vi "PPSU Values 2.vi"(8 "error in":errorcluster, 11 "PPSU 2 Q":refnum<queue>) -> (0 "Fehler":errorcluster caption="Error out")   [LabVIEW 2022 SP3]
uses:
  6D_Global.vi
panel:
  out "Read data 3":string
  out "Read data (hex) 2":u8[](array[numeric]) format="%.0x"
  out "Read data 2":string
  out "Read data (hex)":u8[](array[numeric]) format="%.0x"
  out "Read data":string
  out "array 2":string[](array[string])
  out "match substring":string
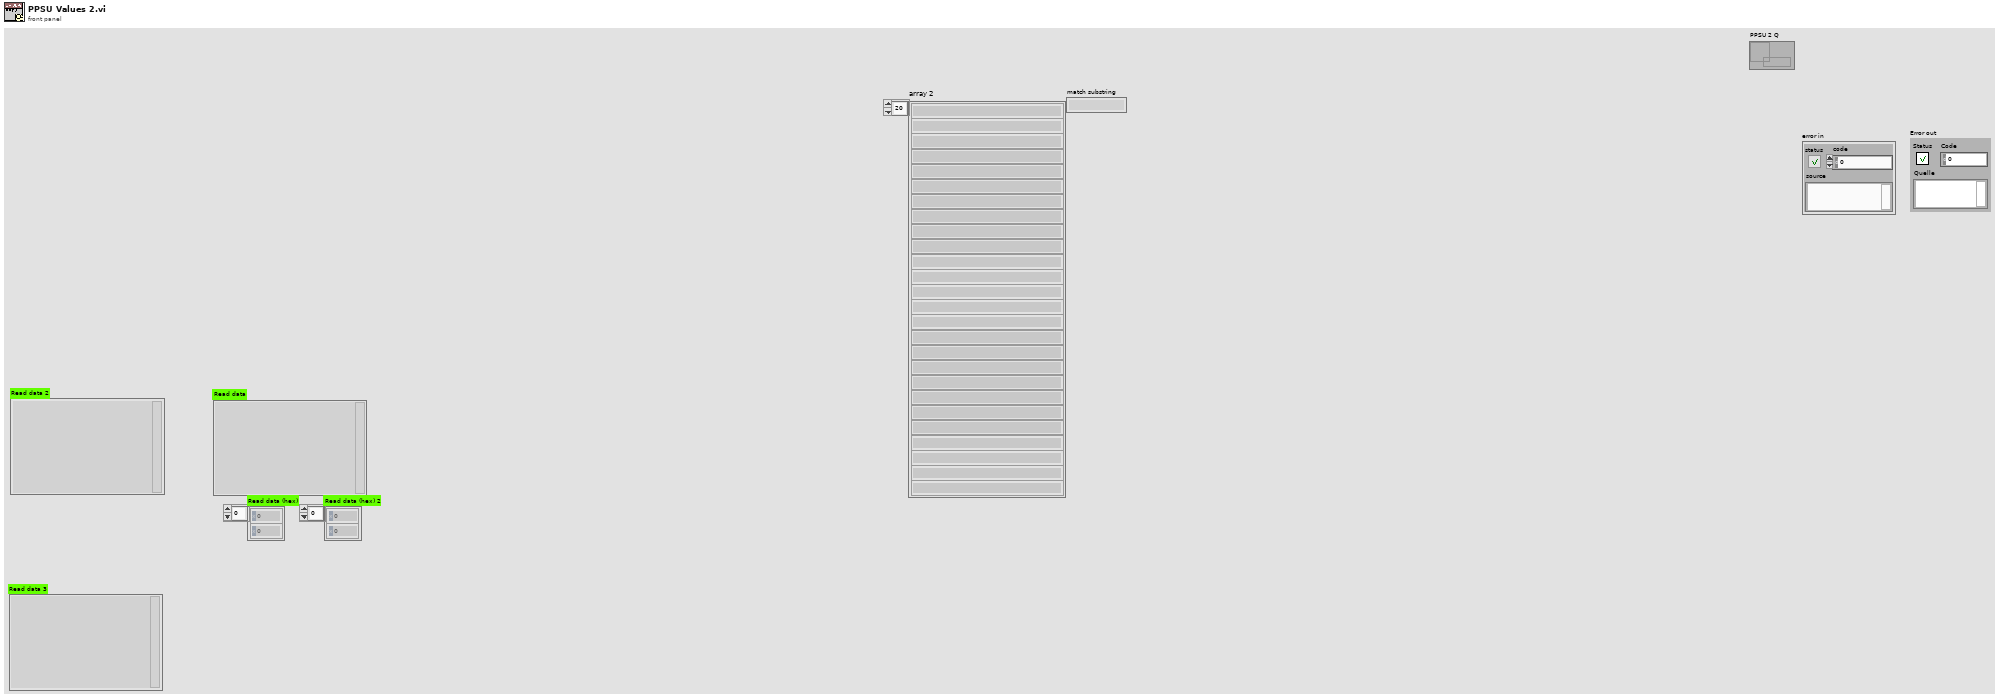
[diagram p1: front panel]
types:
  T1 = cluster{"Alarm":bool, "Power Fail":bool, "OVD":bool, "OCD":bool, "OPD":bool, "MSP":bool}
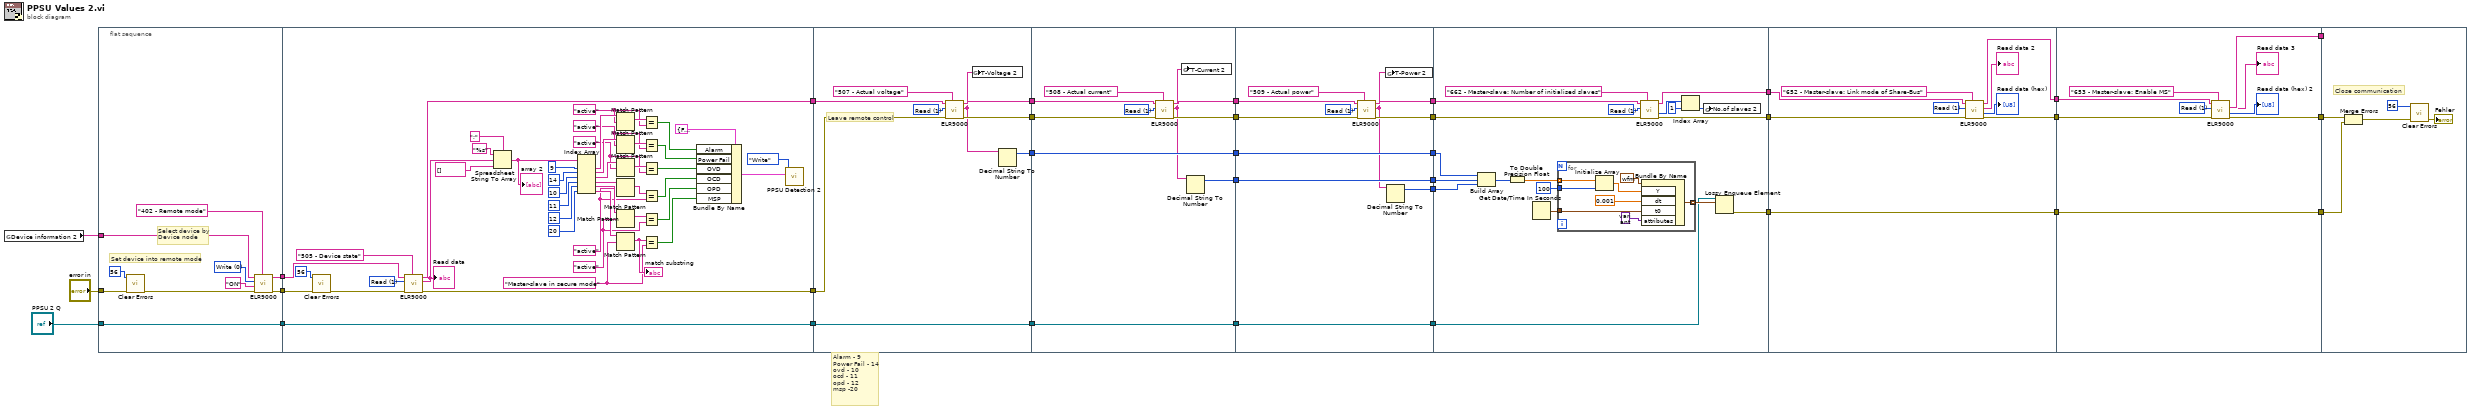
[diagram p0: block diagram]
diagram:
  # "Alarm - 9\nPower Fail - 14\novd - 10\nocd - 11\nopd - 12\nmsp -20"
  n1 = global read "6D_Global.vi" "Device information 2"() -> (w16:string[])
  n2 = flat-sequence {
    tunnel: [w43] -> w32
    tunnel: [w42] -> w33
    tunnel: w16 -> [w38]
    tunnel: "error in" -> [w36]
    tunnel: "PPSU 2 Q" -> [w34]
    tunnel: [w34] -> w14
    tunnel: [w90] -> w31
    tunnel: w33 -> [w87]
    tunnel: w32 -> [w86]
    tunnel: [w55] -> w30
    tunnel: w14 -> [w44]
    tunnel: [w44] -> w13
    tunnel: [w95] -> w29
    tunnel: w31 -> [w97]
    tunnel: [w96] -> w28
    tunnel: w30 -> [w94]
    tunnel: w13 -> [w93]
    tunnel: [w93] -> w12
    tunnel: [w91] -> w9
    tunnel: w29 -> [w105]
    tunnel: [w104] -> w27
    tunnel: w28 -> [w106]
    tunnel: [w107] -> w26
    tunnel: w12 -> [w103]
    tunnel: [w103] -> w11
    tunnel: w9 -> [w102]
    tunnel: [w102] -> w8
    tunnel: [w100] -> w5
    tunnel: w27 -> [w116]
    tunnel: [w115] -> w25
    tunnel: w26 -> [w118]
    tunnel: [w117] -> w24
    tunnel: w11 -> [w114]
    tunnel: [w114] -> w10
    tunnel: w8 -> [w113]
    tunnel: [w113] -> w7
    tunnel: [w112] -> w6
    tunnel: w5 -> [w112]
    tunnel: [w110] -> w4
    tunnel: w25 -> [w137]
    tunnel: [w136] -> w23
    tunnel: w24 -> [w138]
    tunnel: [w139] -> w22
    tunnel: w10 -> [w126]
    tunnel: w7 -> [w125]
    tunnel: w6 -> [w123]
    tunnel: w4 -> [w122]
    tunnel: [w121] -> w3
    tunnel: w23 -> [w154]
    tunnel: [w153] -> w21
    tunnel: w22 -> [w156]
    tunnel: [w155] -> w20
    tunnel: w3 -> [w148]
    tunnel: [w148] -> w2
    tunnel: w21 -> [w163]
    tunnel: [w162] -> w19
    tunnel: w20 -> [w165]
    tunnel: [w164] -> w18
    tunnel: w2 -> [w157]
    tunnel: [w157] -> w1
    tunnel: w19 -> [w170]
    tunnel: w18 -> [_]
    tunnel: w1 -> [w166]
    frame #0 {
      w41 = u8 0 items=["Write", "Read"] ("Access")
      # "Select device by\nDevice node"
      # "Set device into remote mode"
      n3 = call <vilib>:"Clear Errors.vi"("error in (no error)"=w36, "specific error code to clear (0: all)"=56) -> ("error out"=w37:errorcluster)  [unwired: 4 in, 1 out]
      n4 = call <instrlib>:"ELR9000.vi"("Command list"="402 - Remote mode", "Error in"=w37, "Value"="ON", "Access"=w41, "Device information in"=w38) -> ("Error out"=w43:errorcluster, "Device information out"=w42:string[])  [unwired: 1 in, 2 out]
    }
    frame #1 {
      w67 = "Master-slave in secure mode" ("regular expression")
      w54 = "active" ("regular expression")
      w66 = "active" ("regular expression")
      w65 = "active" ("regular expression")
      w64 = "active" ("regular expression")
      w63 = "active" ("regular expression")
      w89 = u8 1 items=["Write", "Read"] ("Access")
      n5 = call <vilib>:"Clear Errors.vi"("error in (no error)"=w86, "specific error code to clear (0: all)"=56) -> ("error out"=w81:errorcluster)  [unwired: 4 in, 1 out]
      n6 = call <instrlib>:"ELR9000.vi"("Command list"="505 - Device state", "Error in"=w81, "Access"=w89, "Device information in"=w87) -> ("Error out"=w55:errorcluster, "Read data"=w85:string, "Device information out"=w90:string[])  [unwired: 2 in, 1 out]
      "Read data" <- w85
      n7 = Spreadsheet String To Array(delimiter (Tab)=";", format string="%s", spreadsheet string=w85, array type (2D Dbl)=string[] []) -> (array=w56:string[])
      "array 2" <- w56
      n8 = Index Array(array=w56, index #1=9 ("index"), index #2=14 ("index"), index #3=10 ("index"), index #4=11 ("index"), index #5=12 ("index"), index #6=20 ("index")) -> (element #1=w74:string, element #2=w75:string, element #3=w76:string, element #4=w77:string, element #5=w78:string, element #6=w79:string)
      n9 = Match Pattern(string=w74, regular expression=w63) -> (match substring=w68:string)  [unwired: 1 in, 3 out]
      n10 = Match Pattern(string=w75, regular expression=w64) -> (match substring=w69:string)  [unwired: 1 in, 3 out]
      n11 = Match Pattern(string=w76, regular expression=w65) -> (match substring=w70:string)  [unwired: 1 in, 3 out]
      n12 = Match Pattern(string=w77, regular expression=w54) -> (match substring=w72:string)  [unwired: 1 in, 3 out]
      n13 = Match Pattern(string=w78, regular expression=w66) -> (match substring=w71:string)  [unwired: 1 in, 3 out]
      n14 = Match Pattern(string=w79, regular expression=w67) -> (match substring=w73:string)  [unwired: 1 in, 3 out]
      "match substring" <- w73
      n15 = Equal?(x=w68, y=w63) -> (x = y?=w52:bool)
      n16 = Equal?(x=w69, y=w64) -> (x = y?=w51:bool)
      n17 = Equal?(x=w70, y=w65) -> (x = y?=w50:bool)
      n18 = Equal?(x=w72, y=w54) -> (x = y?=w49:bool)
      n19 = Equal?(x=w71, y=w66) -> (x = y?=w48:bool)
      n20 = Equal?(x=w73, y=w67) -> (x = y?=w47:bool)
      n21 = Bundle By Name(cluster=T1 {"Alarm"=FALSE, "Power Fail"=FALSE, "OVD"=FALSE, "OCD"=FALSE, "OPD"=FALSE, "MSP"=FALSE} ("PPSU Dect"), "Alarm"=w52, "Power Fail"=w51, "OVD"=w50, "OCD"=w49, "OPD"=w48, "MSP"=w47) -> (w45:T1)
      n22 = call "PPSU Detection 2.vi"("PPSU Dect 2"=w45, "Write/Read"=enum16{"Write", "Read"}."Write") -> ()  [unwired: 8 in, 2 out]
    }
    frame #2 {
      w99 = u8 1 items=["Write", "Read"] ("Access")
      # "Leave remote control"
      n23 = call <instrlib>:"ELR9000.vi"("Command list"="507 - Actual voltage", "Error in"=w94, "Access"=w99, "Device information in"=w97) -> ("Error out"=w95:errorcluster, "Read data"=w92:string, "Device information out"=w96:string[])  [unwired: 2 in, 1 out]
      n24 = global write "6D_Global.vi" "T-Voltage 2"(w92) -> ()
      n25 = Decimal String To Number(string=w92) -> (offset past number=w91:i32)  [unwired: 2 in, 1 out]
    }
    frame #3 {
      w108 = u8 1 items=["Write", "Read"] ("Access")
      n26 = call <instrlib>:"ELR9000.vi"("Command list"="508 - Actual current", "Error in"=w105, "Access"=w108, "Device information in"=w106) -> ("Error out"=w104:errorcluster, "Read data"=w101:string, "Device information out"=w107:string[])  [unwired: 2 in, 1 out]
      n27 = global write "6D_Global.vi" "T-Current 2"(w101) -> ()
      n28 = Decimal String To Number(string=w101) -> (offset past number=w100:i32)  [unwired: 2 in, 1 out]
    }
    frame #4 {
      w120 = u8 1 items=["Write", "Read"] ("Access")
      n29 = call <instrlib>:"ELR9000.vi"("Command list"="509 - Actual power", "Error in"=w116, "Access"=w120, "Device information in"=w118) -> ("Error out"=w115:errorcluster, "Read data"=w111:string, "Device information out"=w117:string[])  [unwired: 2 in, 1 out]
      n30 = global write "6D_Global.vi" "T-Power 2"(w111) -> ()
      n31 = Decimal String To Number(string=w111) -> (offset past number=w110:i32)  [unwired: 2 in, 1 out]
    }
    frame #5 {
      w134 = u8 1 items=["Write", "Read"] ("Access")
      n32 = Build Array(w125, w123, w122) -> (w124:i32[])
      n33 = To Double Precision Float(number=w124) -> (double precision float=w127:dbl[])
      n34 = Get Date/Time In Seconds() -> (seconds since 1Jan1904=w129:timestamp)
      n35 = for {
        tunnel: w127 -> [w147] mode=indexing
        tunnel: 100 ("dimension size") -> [w146]
        tunnel: [w142] -> w130 mode=indexing
        tunnel: w129 -> [w140]
        n36 = Initialize Array(w147, w146) -> (w145:dbl[])
        n37 = Bundle By Name(cluster=waveform(dbl) {"t0"=timestamp(0 s since 1904-01-01), "dt"=1.0, "Y"=[]} ("waveform"), "Y"=w145, "dt"=0.001, "t0"=w140, "attributes"=variant) -> (w142:waveform(dbl))
      }
      n38 = call <instrlib>:"ELR9000.vi"("Command list"="662 - Master-slave: Number of initialised slaves", "Error in"=w137, "Access"=w134, "Device information in"=w138) -> ("Error out"=w136:errorcluster, "Read data (hex)"=w133:u8[], "Device information out"=w139:string[])  [unwired: 2 in, 1 out]
      n39 = Index Array(array=w133, index=1) -> (element=w131:u8)
      n40 = global write "6D_Global.vi" "No.of slaves 2"(w131) -> ()
      n41 = Lossy Enqueue Element(queue=w126, element=w130) -> (error out=w121:errorcluster)  [unwired: 1 in, 3 out]
    }
    frame #6 {
      w152 = u8 1 items=["Write", "Read"] ("Access")
      n42 = call <instrlib>:"ELR9000.vi"("Command list"="652 - Master-slave: Link mode of Share-Bus", "Error in"=w154, "Access"=w152, "Device information in"=w156) -> ("Error out"=w153:errorcluster, "Read data (hex)"=→"Read data (hex)":u8[], "Read data"=→"Read data 2":string, "Device information out"=w155:string[])  [unwired: 2 in]
    }
    frame #7 {
      w161 = u8 1 items=["Write", "Read"] ("Access")
      n43 = call <instrlib>:"ELR9000.vi"("Command list"="653 - Master-slave: Enable MS", "Error in"=w163, "Access"=w161, "Device information in"=w165) -> ("Error out"=w162:errorcluster, "Read data (hex)"=→"Read data (hex) 2":u8[], "Read data"=→"Read data 3":string, "Device information out"=w164:string[])  [unwired: 2 in]
    }
    frame #8 {
      # "Close communication"
      n44 = Merge Errors(w170, w166) -> (w167:errorcluster)
      n45 = call <vilib>:"Clear Errors.vi"("error in (no error)"=w167, "specific error code to clear (0: all)"=56) -> ("error out"=→"Fehler":errorcluster)  [unwired: 4 in, 1 out]
    }
  }
